vi "Variant to SGL.vi"(2 "Variant":variant) -> (7 "Value":sgl)   [LabVIEW 2021, in "Variant to Data.lvlib"]
uses:
  Variant to Data.lvlib
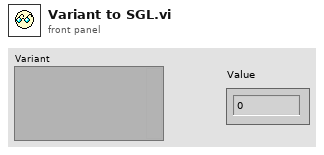
[diagram p1: front panel]
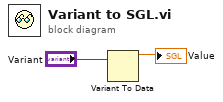
[diagram p0: block diagram]
diagram:
  n1 = Variant To Data(Variant="Variant") -> (data=→"Value":sgl)  [unwired: 2 in, 1 out]
